vi "题目3.vi"() -> ()   [LabVIEW 2017]
panel:
  out "数组":dbl[][](array[numeric])
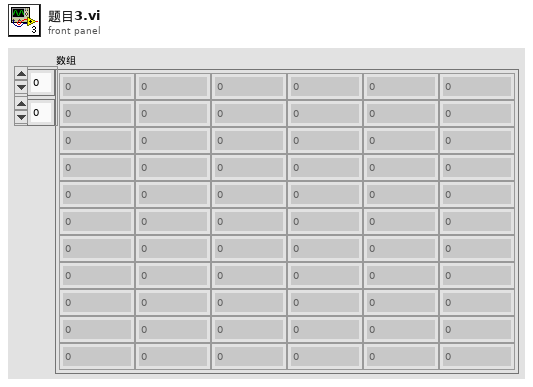
[diagram p1: front panel]
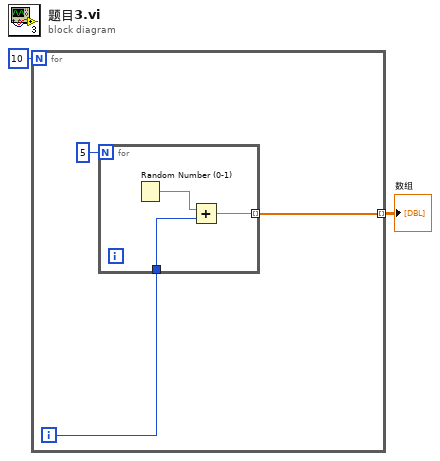
[diagram p0: block diagram]
diagram:
  n1 = for {
    N: 10 -> [_]
    tunnel: [w4] -> w1 mode=indexing
    i -> [w3]
    n2 = for {
      N: 5 -> [_]
      tunnel: [w7] -> w4 mode=indexing
      tunnel: w3 -> [w6]
      n3 = Random Number (0-1)() -> (number: 0 to 1=w8:dbl)
      n4 = Add(x=w8, y=w6) -> (x+y=w7:dbl)
    }
  }
  "数组" <- w1
